vi "folder recrusive.vi"(11 "path":path) -> (3 "Array":path[](array[path]))   [LabVIEW 2023]
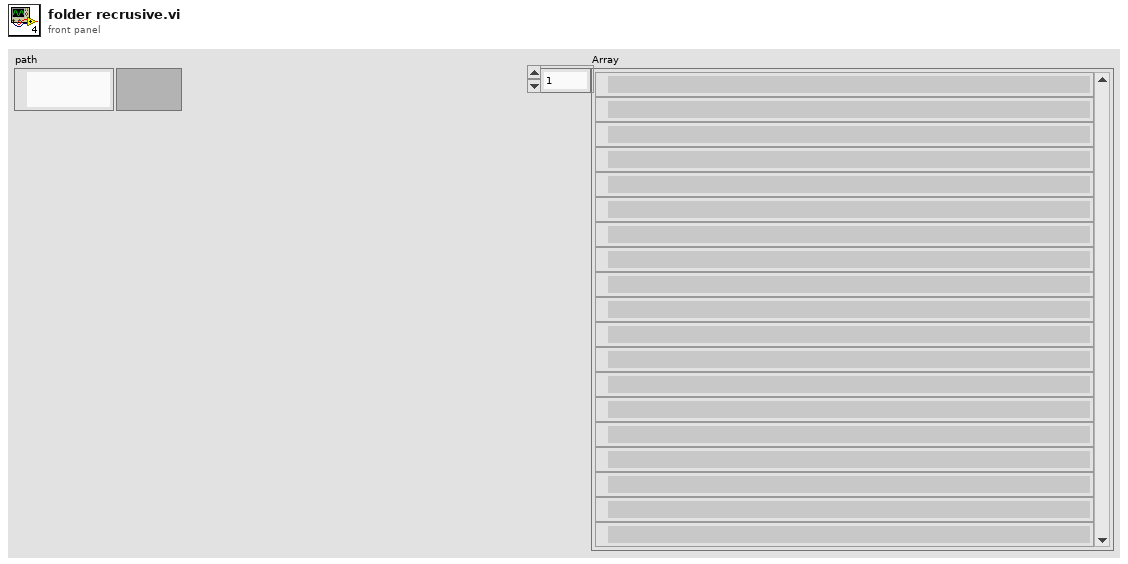
[diagram p1: front panel]
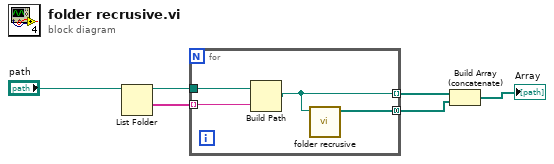
[diagram p0: block diagram]
diagram:
  n1 = List Folder(path="path") -> (path out=w2:path, folder names=w5:string[])  [unwired: 2 in, 3 out]
  n2 = for {
    tunnel: w2 -> [w10]
    tunnel: w5 -> [w9] mode=indexing
    tunnel: [w8] -> w4 mode=indexing
    tunnel: [w7] -> w1 mode=concatenating
    n3 = Build Path(base path=w10, name or relative path=w9) -> (appended path=w8:path)
    n4 = call "folder recrusive.vi"("path"=w8) -> ("Array"=w7:path[])  [unwired: 10 in]
  }
  n5 = Build Array (concatenate)(w4, w1) -> (→"Array":path[])
